vi "AdjustableVoltage.vi"() -> ()   [LabVIEW 2015]
uses:
  <vilib>/DAQmx/write.llb/DAQmx Write (Analog DBL 1Chan 1Samp).vi
  <vilib>/DAQmx/miscellaneous.llb/DAQmx Fill In Error Info.vi
panel:
  in  "task/channels in":refnum<k21>="IamA1"
  in  "Voltage (red)":dbl(knob) min=0.0 step=0.1 scale=0.0..5.0
  in  "Stop Button":bool
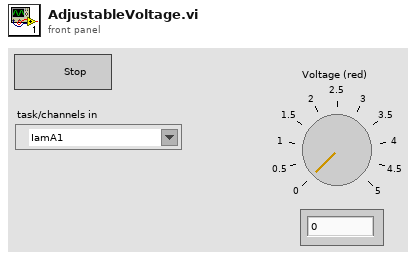
[diagram p1: front panel]
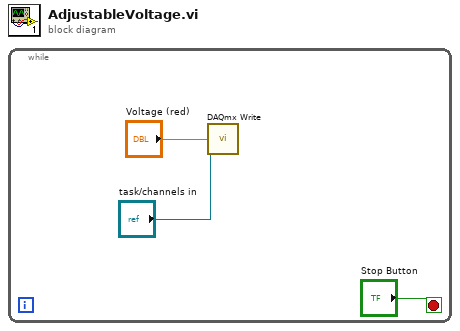
[diagram p0: block diagram]
diagram:
  n1 = while {
    stop <- "Stop Button" stop-if-true
    n2 = call-poly <vilib>:"DAQmx Write.vi"("task/channels in"="task/channels in", "data"="Voltage (red)") -> ()  [unwired: 11 in, 3 out]
  }
